vi "stage_load.vi"(4 "image array":T1[](array[typedef]), 5 "map file":path) -> (0 "hum_pos":cluster{"pos.x":i32, "pos.y":i32}, 1 "picture":picture, 2 "status array":u8[][](array[numeric]))   [LabVIEW 2018]
uses:
  <vilib>/picture/picture.llb/imagedata.ctl
  examples/LABVIEW Boxman/boxman1.03.llb/global.vi
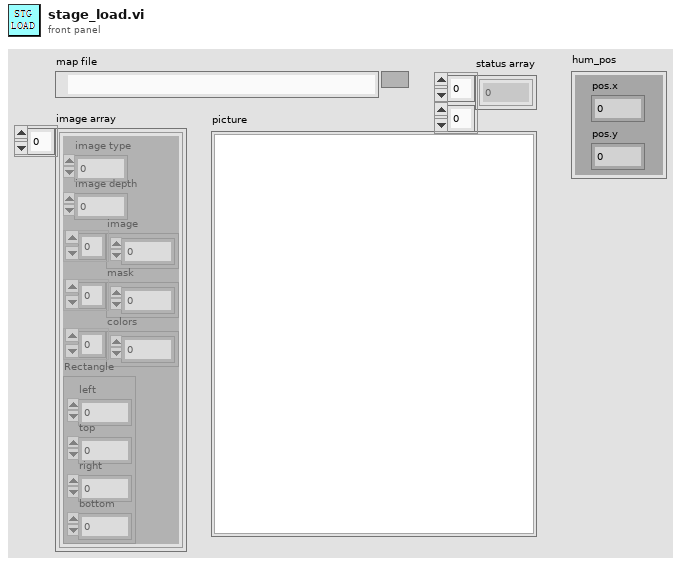
[diagram p1: front panel]
types:
  T1 = typedef "imagedata.ctl" = cluster{"image type":i32, "image depth":i32, "image":u8[], "mask":u8[], "colors":u32[], "Rectangle":cluster{"left":i16, "top":i16, "right":i16, "bottom":i16}}
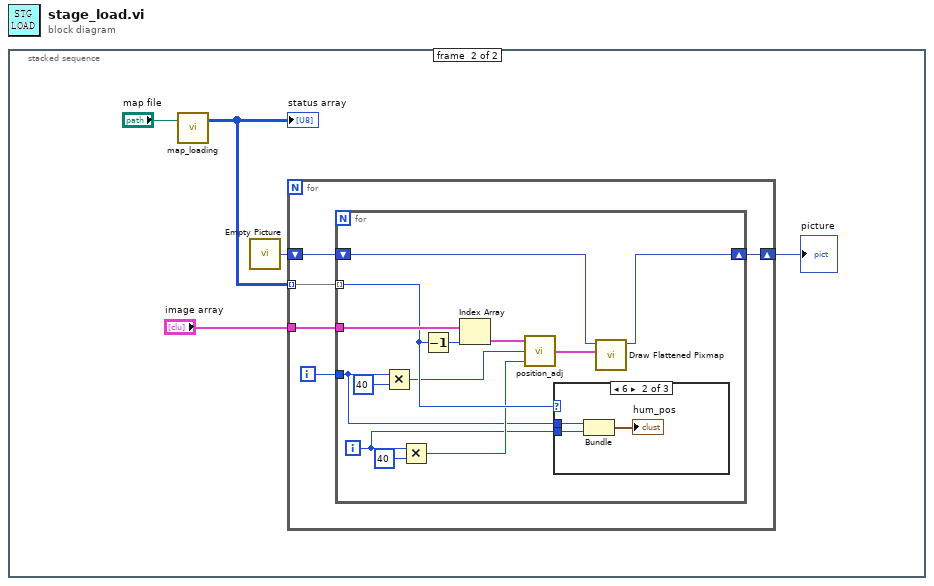
[diagram p0: block diagram]
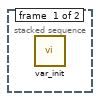
[diagram p2: hidden frame]
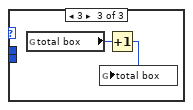
[diagram p4: hidden frame]
diagram:
  n1 = stacked-sequence {
    frame #0 {
      n2 = call "var_init.vi"() -> ()  [unwired: 12 in]
    }
    frame #1 {
      n3 = call "map_loading.vi"("map file"="map file") -> ("status array"=w1:u8[][])  [unwired: 2 in]
      "status array" <- w1
      n4 = call "Empty Picture"() -> ("empty picture"=w5:picture)
      n5 = for {
        tunnel: w1 -> [w10] mode=indexing
        tunnel: "image array" -> [w9]
        shift-right: [w6] -> w4
        shift-left: w5 -> [w8]
        i -> [w7]
        n6 = for {
          tunnel: w10 -> [w15] mode=indexing
          tunnel: w9 -> [w23]
          shift-right: [w17] -> w6
          shift-left: w8 -> [w22]
          tunnel: w7 -> [w12]
          i -> [w11]
          n7 = Multiply(x=w12, y=u32 40) -> (x*y=w14:u32)
          n8 = Multiply(x=w11, y=u32 40) -> (x*y=w13:u32)
          n9 = Decrement(x=w15) -> (x-1=w16:u8)
          n10 = Index Array(array=w23, index=w16) -> (element=w21:T1)
          n11 = call "position_adj.vi"("coordinate.y"=w13, "coordinate.x"=w14, "image data in"=w21) -> ("image data out"=w18:T1)
          n12 = case shown="6" w15 {
            tunnel: w12 -> [_ w26 _]
            tunnel: w11 -> [_ w25 _]
            frame Default {
            }
            frame 6 {
              n13 = Bundle(w26, w25) -> (→"hum_pos":cluster{i32, i32})  [unwired: 1 in]
            }
            frame 3 {
              n14 = global read "global.vi" "total box"() -> (w27:u32)
              n15 = Increment(x=w27) -> (x+1=w28:u32)
              n16 = global write "global.vi" "total box"(w28) -> ()
            }
          }
          n17 = call <vilib>:"Draw Flattened Pixmap.vi"("image data"=w18, "picture"=w22) -> ("new picture"=w17:picture)  [unwired: 7 in]
        }
      }
      "picture" <- w4
    }
  }
